vi "SSL Detection Frame Robots Kalman Estimator VelCmd.vi"(0 "Lado":enum16{"Esquerdo", "Direito"}(ring) caption="Enum", 5 "Time Stamp":timestamp, 6 "our_robots":bool=TRUE, 7 "Life Time":dbl=1.0, 8 "ignora esquerda?":bool, 9 "ignora lado":bool, 10 "our_robots":T1[](array[typedef]), 11 "Robots":T6[](array[typedef]) {"height" format="%+4.3f"; "pixel_y" format="%+4.3f"; "pixel_x" format="%+4.3f"; "orientation" format="%+4.3f"; "y" format="%+4.3f"; "confidence" format="%4.3f"; "x" format="%+4.3f"}) -> (3 "Robots Out":T6[](array[typedef]) {"height" format="%+4.3f"; "pixel_y" format="%+4.3f"; "pixel_x" format="%+4.3f"; "orientation" format="%+4.3f"; "y" format="%+4.3f"; "confidence" format="%4.3f"; "x" format="%+4.3f"})   [LabVIEW 2018]
uses:
  SSL Detection Robot.ctl
  <vilib>/Analysis/Matrix/Datatypes/RealMatrix.ctl
  Core/AI Robot.ctl
  Intel/Functions Enum.ctl
  Intel/AttackerStates.ctl
  Path Planning/RRT/PathDests.ctl
  Path Planning/RRT/PathDest.ctl
  <vilib>/Analysis/coordinate.llb/Wrap Angle (scalar).vi
  <vilib>/Analysis/_algsub.llb/Real Vector Norm.vi
  <vilib>/Analysis/Matrix/Numeric/Conversions/Array To Matrix - RA.vi
  <vilib>/Analysis/Matrix/Numeric/Subtract/Subtract - RM,RM.vi
  <vilib>/Analysis/NI_AALPro.lvlib
  <vilib>/Analysis/Matrix/NI_Matrix.lvlib
  <vilib>/Analysis/NI_AAL_Angle.lvlib
panel:
  in  "Robots Out 2":T8(array[cluster]) {"Detection Robot"."height" format="%+4.3f"; "Detection Robot"."pixel_y" format="%+4.3f"; "Detection Robot"."pixel_x" format="%+4.3f"; "Detection Robot"."orientation" format="%+4.3f"; "Detection Robot"."y" format="%+4.3f"; "Detection Robot"."confidence" format="%4.3f"; "Detection Robot"."x" format="%+4.3f"}
  out "A-B":dbl[][](array[numeric])
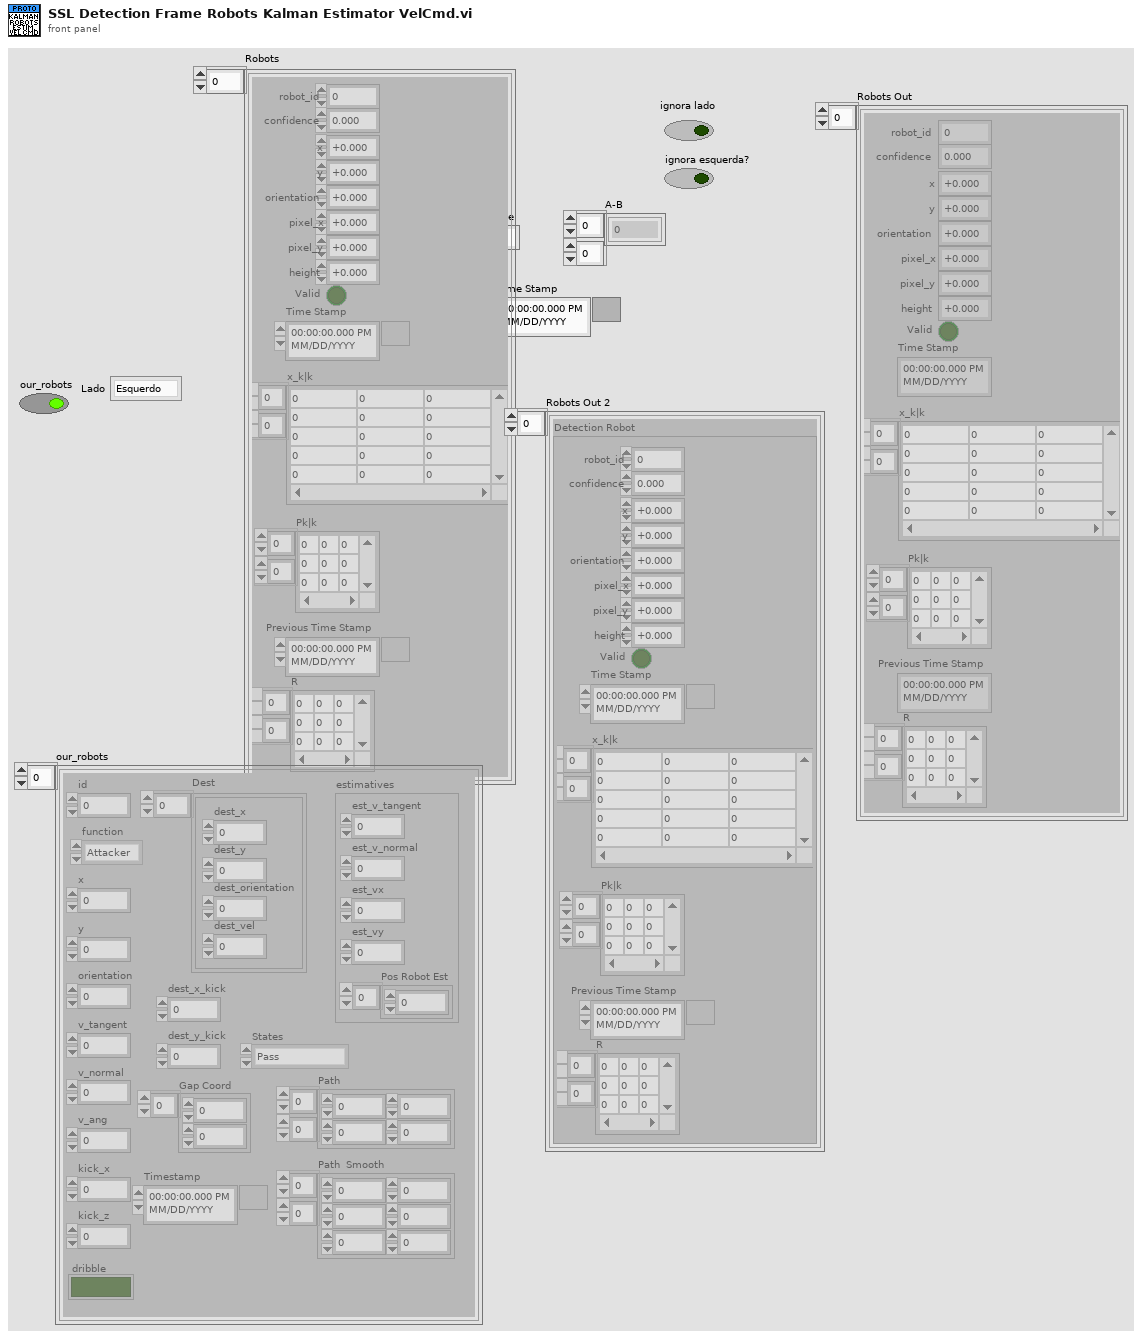
[diagram p1: front panel]
types:
  T1 = typedef "AI Robot.ctl" = cluster{"id":u32, "function":T2, "x":dbl, "y":dbl, "orientation":dbl, "v_tangent":dbl, "v_normal":dbl, "v_ang":dbl, "kick_x":dbl, "kick_z":dbl, "dribble":bool, "Timestamp":timestamp, "estimatives":cluster{"est_v_tangent":dbl, "est_v_normal":dbl, "est_vx":dbl, "est_vy":dbl, "Pos Robot Est":dbl[]}, "dest_x_kick":dbl, "dest_y_kick":dbl, "Gap Coord":dbl[], "States":T3, "Path ":dbl[][], "Path  Smooth":dbl[][], "Dest":T4}
  T2 = typedef "Functions Enum.ctl" = enum16{"2nd Striker", "Attacker", "Goalie", "Defender", "Striker", "Goto 0", "Dummy", "Kicker", "ZigZag 0", "ZigZag 1", "ZigZag 2", "ZigZag 3", "ZigZag 4", "ZigZag 5", "ZigZag 6", "ZigZag 7", "ZigZag 8", ""}
  T3 = typedef "AttackerStates.ctl" = enum16{"Pass", "GoToTangent", "BallGetting", "GoToKick", ""}
  T4 = typedef "PathDests.ctl" = T5[]
  T5 = typedef "PathDest.ctl" = cluster{"dest_x":dbl, "dest_y":dbl, "dest_orientation":dbl, "dest_vel":dbl}
  T6 = typedef "SSL Detection Robot.ctl" = cluster{"x":sgl, "robot_id":u32, "confidence":sgl, "y":sgl, "orientation":sgl, "pixel_x":sgl, "pixel_y":sgl, "height":sgl, "Valid":bool, "Time Stamp":timestamp, "x_k|k":T7, "Pk|k":T7, "Previous Time Stamp":timestamp, "R":T7}
  T7 = typedef "NI_Matrix.lvlib/RealMatrix.ctl" = dbl[][]
  T8 = cluster{"Detection Robot":T6, "Real Matrix (Column Vector)":T7, "Pk|k":T7}[]
  T9 = cluster{"Detection Robot":T6, "Real Matrix (Column Vector)":T7, "Pk|k":T7}
  T10 = cluster{"Detection Robot out":T6, "x_k|k":T7, "Pk|k":T7}
  T11 = typedef "SSL Detection Robot.ctl" = cluster{"x":sgl, "robot_id":u32, "confidence":sgl, "y":sgl, "orientation":sgl, "pixel_x":sgl, "pixel_y":sgl, "height":sgl, "Valid":bool, "Time Stamp":timestamp, "x_k|k":T7, "Pk|k":T7}
  T12 = cluster{"Detection Robot":T11, "Real Matrix (Column Vector)":T7, dbl[][]}
  T13 = cluster{"Detection Robot out":T6, "x_k|k":T7, "Pk|k":T7}[]
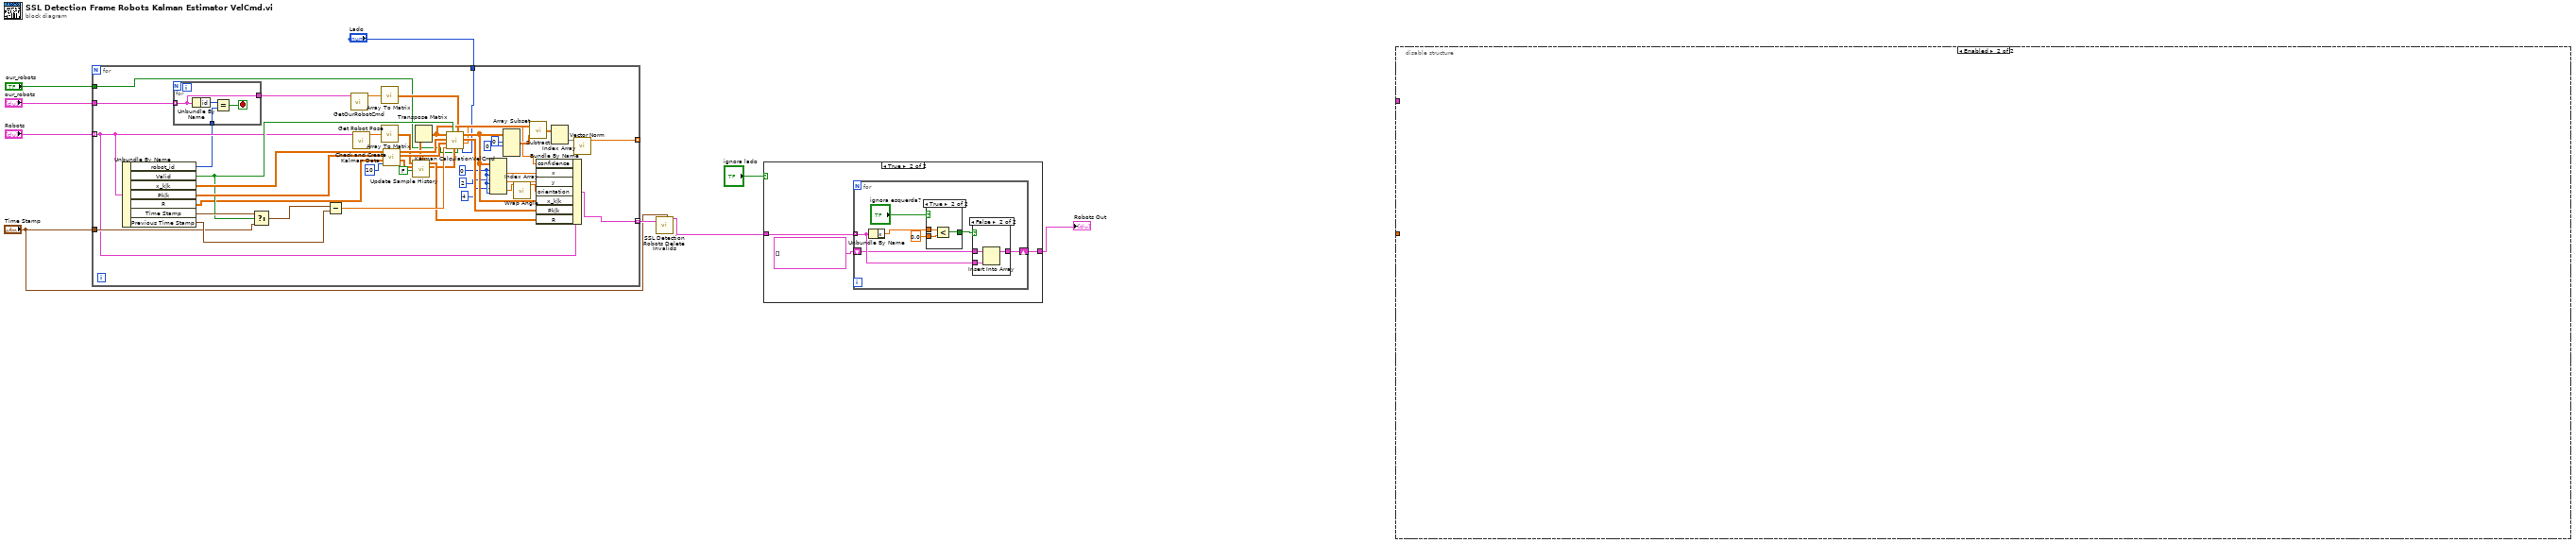
[diagram p0: block diagram]
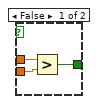
[diagram p3: hidden frame]
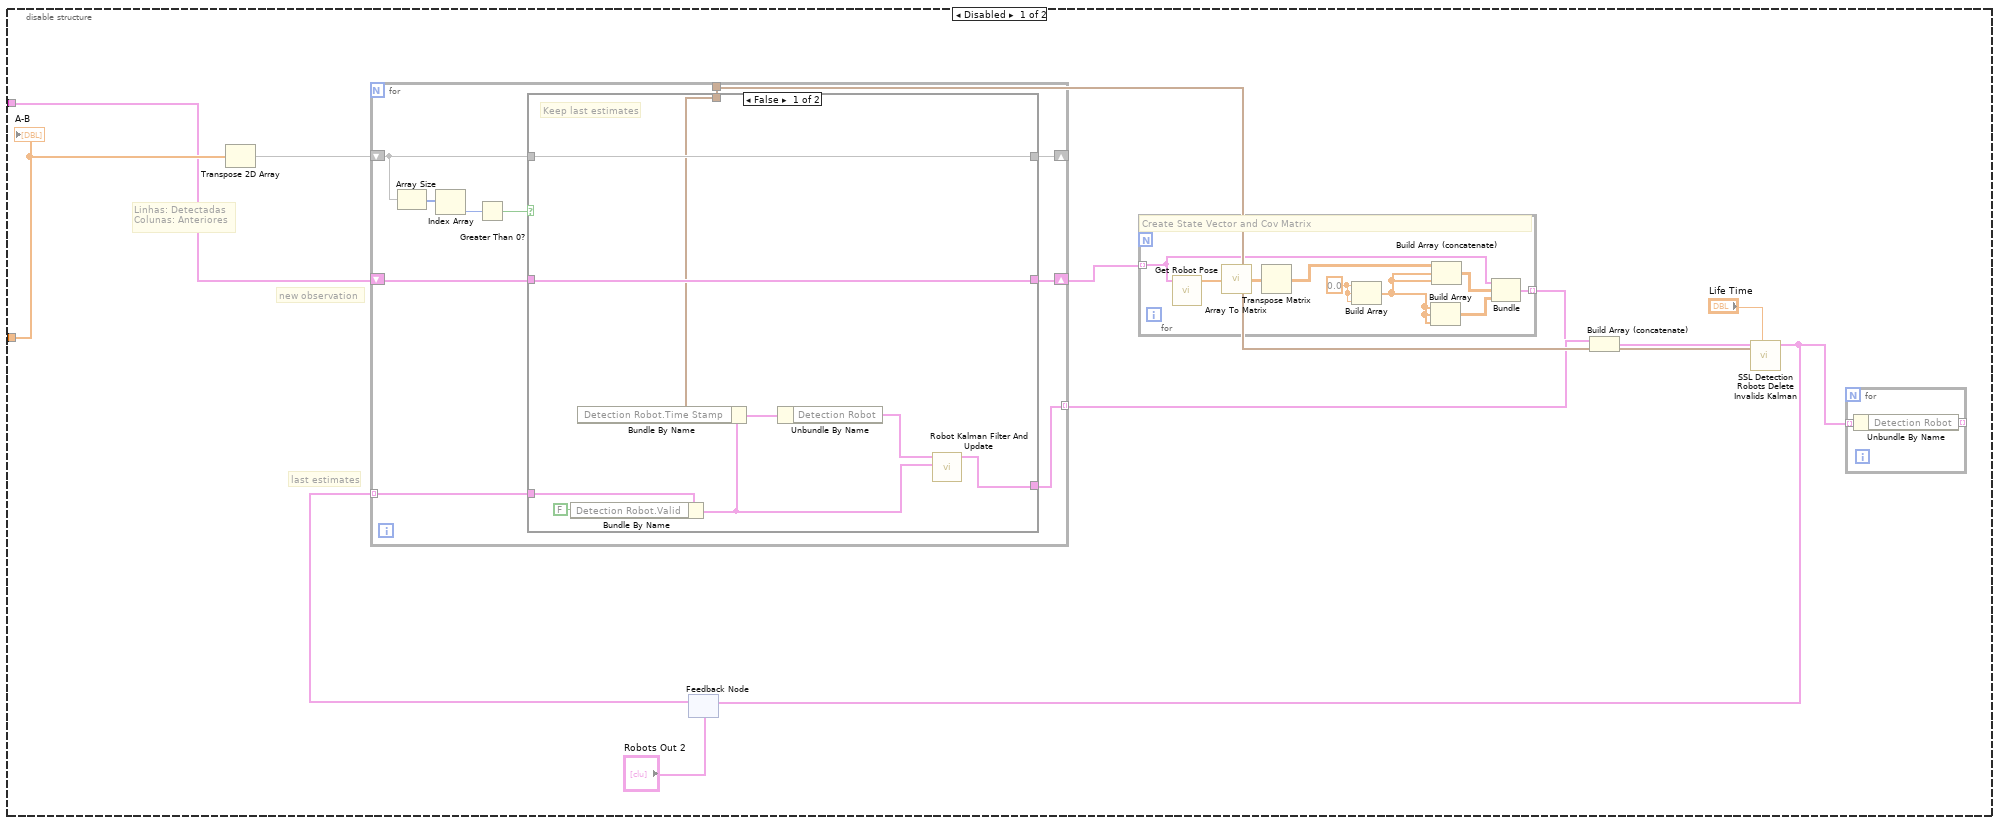
[diagram p5: hidden frame]
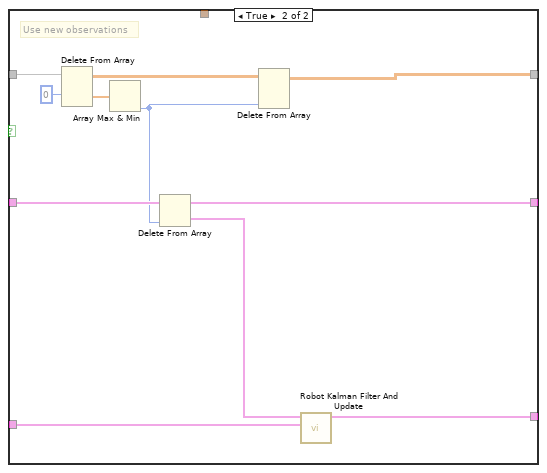
[diagram p6: hidden frame]
diagram:
  n1 = for {
    tunnel: "Robots" -> [w36] mode=indexing
    tunnel: [w54] -> _ mode=indexing
    tunnel: [w18] -> w8 mode=indexing
    tunnel: "Time Stamp" -> [w39]
    tunnel: "our_robots" -> [w17]
    tunnel: "our_robots" -> [w12]
    tunnel: "Lado" -> [w11]
    w32 = 0 ("index (row)")
    n2 = Unbundle By Name(w36) -> ("robot_id"=w16:u32, "Valid"=w37:bool, "x_k|k"=w46:T7, "Pk|k"=w44:T7, "R"=w29:T7, "Time Stamp"=w40:timestamp, "Previous Time Stamp"=w42:timestamp)
    n3 = for {
      tunnel: w17 -> [w55] mode=indexing
      tunnel: w16 -> [w56]
      tunnel: [w55] -> w15
      stop <- w58 stop-if-true
      n4 = Unbundle By Name(w55) -> ("id"=w57:u32)
      n5 = Equal?(x=w57, y=w56) -> (x = y?=w58:bool)
    }
    n6 = Select(t=w40, s=w37, f=w39) -> (s? t:f=w38:timestamp)
    n7 = Subtract(x=w38, y=w42) -> (x-y=w41:dbl)
    n8 = call "GetOurRobotCmd.vi"("Robot"=w15) -> ("Vel"=w14:dbl[])  [unwired: 10 in]
    n9 = call "Get Robot Pose.vi"("Detection Robot"=w36) -> ("Pose"=w48:sgl[])  [unwired: 10 in]
    n10 = call-poly <vilib>:"Array To Matrix.vi"("Real 1D Array"=w14) -> ("Real Matrix (Column Vector)"=w13:T7)
    n11 = call-poly <vilib>:"Array To Matrix.vi"("Real 1D Array"=w48) -> ("Real Matrix (Column Vector)"=w25:T7)
    n12 = call "Check and Create Kalman Data.vi"("Variance Memory"=10, "R"=w29, "Pk"=w44, "x_k"=w46) -> ("R out"=w28:T7, "Pk out"=w43:T7, "x_k out"=w45:T7)  [unwired: 5 in]
    n13 = call "Update Sample History.vi"("Ball?"=FALSE, "R in"=w28, "Sample"=w25) -> ("covariance matrix V"=w23:T7, "R out"=w24:T7, "Sample Unwrapped"=w22:T7)  [unwired: 6 in]
    n14 = Transpose Matrix(1:w22) -> (0:w26:T7)
    n15 = call "Kalman CalculationVelCmd.vi"("Lado"=w11, "our_robots"=w12, "u_k"=w13, "R"=w23, "Use Observation"=w37, "intervalo"=w41, "Pk-1|k-1"=w43, "x_k-1|k-1"=w45, "z_k"=w26) -> ("Conf"=w19:dbl, "Pk|k"=w47:T7, "x_k|k"=w35:T7)
    n16 = Index Array(array=w35, index (row) #1=w32, index (col) #1=w32, index (row) #2=2 ("disabled index (col)"), index (col) #2=w32, index (row) #3=4 ("disabled index (col)"), index (col) #3=w32) -> (element #1=w34:dbl, element #2=w33:dbl, element #3=w21:dbl)
    n17 = Array Subset(array=w35, index (row)=0 ("row 1"), length (row)=0 ("row N")) -> (w53:T7)  [unwired: 2 in]
    n18 = call-poly <vilib>:"Wrap Angle.vi"("angle in"=w21) -> ("angle out"=w20:dbl)  [unwired: 9 in, 1 out]
    n19 = call-poly <vilib>:"Subtract.vi"("Real Matrix B"=w53, "Real Matrix A"=w26) -> ("A - B"=w50:T7)
    n20 = Bundle By Name(cluster=w36, "confidence"=w19, "x"=w34, "y"=w33, "orientation"=w20, "x_k|k"=w35, "Pk|k"=w47, "R"=w24) -> (w18:T6)
    n21 = Index Array(array=w50) -> (element=w49:dbl[])  [unwired: 2 in]
    n22 = call-poly <vilib>:"Vector Norm.vi"("Input Vector"=w49) -> ("norm"=w54:dbl)  [unwired: 9 in, 1 out]
  }
  n23 = call "SSL Detection Robots Delete Invalids.vi"("Now"="Time Stamp", "Robots In"=w8) -> ("Robots Out"=w5:T6[])  [unwired: 9 in]
  n24 = case shown="True" "ignora lado" {
    tunnel: w5 -> [w59 w62]
    tunnel: [w59 w60] -> w4
    frame False {
    }
    frame True {
      n25 = for {
        tunnel: w62 -> [w69] mode=indexing
        shift-right: [w63] -> w60
        shift-left: T6[] [] ("Robots Out") -> [w64]
        n26 = Unbundle By Name(w69) -> ("x"=w68:sgl)
        n27 = case shown="True" "ignora esquerda?" {
          tunnel: w68 -> [w72 w75]
          tunnel: sgl 0.0 ("y") -> [w71 w74]
          tunnel: [w70 w73] -> w66
          frame False {
            n28 = Greater?(x=w72, y=w71) -> (0:w70:bool)
          }
          frame True {
            n29 = Less?(x=w75, y=w74) -> (x < y?=w73:bool)
          }
        }
        n30 = case shown="False" w66 {
          tunnel: w69 -> [_ w78]
          tunnel: [w76 w79] -> w63
          tunnel: w64 -> [w76 w77]
          frame True {
          }
          frame False {
            n31 = Insert Into Array(array=w77, new element=w78) -> (w79:T6[])  [unwired: 1 in]
          }
        }
      }
    }
  }
  "Robots Out" <- w4
  n32 = disable-structure shown="Enabled" {
    disable-tunnel: _ -> [w88 _]
    disable-tunnel: _ -> [w87 _]
    frame Disabled {
      # "Linhas: Detectadas\nColunas: Anteriores"
      # "last estimates"
      # "new observation"
      n33 = Transpose 2D Array(2D array=w88) -> (transposed array=w89:dbl[][])
      n34 = feedback #1("Robots Out 2") -> (w81:T8)
      n35 = for {
        shift-right: [w111] -> _
        shift-left: w89 -> [w107]
        shift-right: [w110] -> w86
        shift-left: w87 -> [w112]
        tunnel: [w109] -> w85 mode=indexing
        tunnel: w81 -> [w108] mode=indexing
        tunnel: [w103] -> w90
        n36 = Array Size(array=w107) -> (size(s)=w105:i32[])
        n37 = Index Array(array=w105) -> (element=w104:i32)  [unwired: 1 in]
        n38 = Greater Than 0?(x=w104) -> (x > 0?=w106:bool)
        n39 = case shown="False" w106 {
          tunnel: w107 -> [w121 w132]
          tunnel: w112 -> [w120 w129]
          tunnel: [w121 w127] -> w111
          tunnel: [w120 w125] -> w110
          tunnel: [w116 w124] -> w109
          tunnel: w108 -> [w115 w122]
          tunnel: w103 -> [w118 _]
          frame False {
            # "Keep last estimates"
            n40 = Bundle By Name(cluster=w115, "Detection Robot.Valid"=FALSE ("Detection Ball.Valid")) -> (w113:T9)
            n41 = Bundle By Name(cluster=w113, "Detection Robot.Time Stamp"=w118) -> (w117:T9)
            n42 = Unbundle By Name(w117) -> ("Detection Robot"=w114:T6)
            n43 = call "Robot Kalman Filter And Update.vi"("Cluster in"=w113, "Detection Robot"=w114) -> ("Cluster out"=w116:T10)  [unwired: 9 in]
          }
          frame True {
            # "Use new observations"
            n44 = Delete From Array(array=w132, index (row)=0) -> (deleted portion=w130:dbl[], array with subset deleted=w128:dbl[][])  [unwired: 2 in]
            n45 = Array Max & Min(array=w130) -> (min index (indices)=w126:i32)  [unwired: 3 out]
            n46 = Delete From Array(array=w129, index=w126) -> (deleted portion=w123:T11, array with subset deleted=w125:T11[])  [unwired: 1 in]
            n47 = Delete From Array(array=w128, index (col)=w126) -> (array with subset deleted=w127:dbl[][])  [unwired: 2 in, 1 out]
            n48 = call "Robot Kalman Filter And Update.vi"("Cluster in"=w122, "Detection Robot"=w123) -> ("Cluster out"=w124:T10)  [unwired: 9 in]
          }
        }
      }
      n49 = for {
        tunnel: w86 -> [w95] mode=indexing
        tunnel: [w98] -> w84 mode=indexing
        w102 = 0.0 ("element")
        # "Create State Vector and Cov Matrix"
        n50 = call "Get Robot Pose.vi"("Detection Robot"=w95) -> ("Pose"=w97:sgl[])  [unwired: 10 in]
        n51 = call-poly <vilib>:"Array To Matrix.vi"("Real 1D Array"=w97) -> ("Real Matrix (Column Vector)"=w96:T7)
        n52 = Transpose Matrix(1:w96) -> (0:w94:T7)
        n53 = Build Array(w102, w102, w102) -> (w101:dbl[])
        n54 = Build Array(w101, w101, w101) -> (w100:dbl[][])
        n55 = Build Array (concatenate)(w94, w101, w101) -> (w99:T7)
        n56 = Bundle("Detection Robot"=w95, "Real Matrix (Column Vector)"=w99, w100) -> (w98:T12)  [unwired: 1 in]
      }
      n57 = Build Array (concatenate)(w85, w84) -> (w80:T13)
      n58 = call "SSL Detection Robots Delete Invalids Kalman.vi"("Now"=w90, "Life Time"="Life Time", "Robots In"=w80) -> ("Robots Out"=w83:T8)  [unwired: 8 in]
      n59 = feedback-in #1(w83) -> ()
      n60 = for {
        tunnel: w83 -> [w93] mode=indexing
        tunnel: [w92] -> _ mode=indexing
        n61 = Unbundle By Name(w93) -> ("Detection Robot"=w92:T6)
      }
      "A-B" <- w88
    }
    frame Enabled {
    }
  }
